vi "SpinProgramCheck.vi"() -> ()   [LabVIEW 2018]
uses:
  <instrlib>/Classes/SpinCoater/SpinCoater.lvclass
panel:
  out "Spin Program":dbl[][](array[numeric])
  in  "Time Start":dbl[unit]
  in  "Program":dbl[][](array[numeric])
  out "Init":bool
  in  "VISA resource name":refnum<visa-resource-name>
  in  "Cancel Button":bool
  out "Time Left":dbl
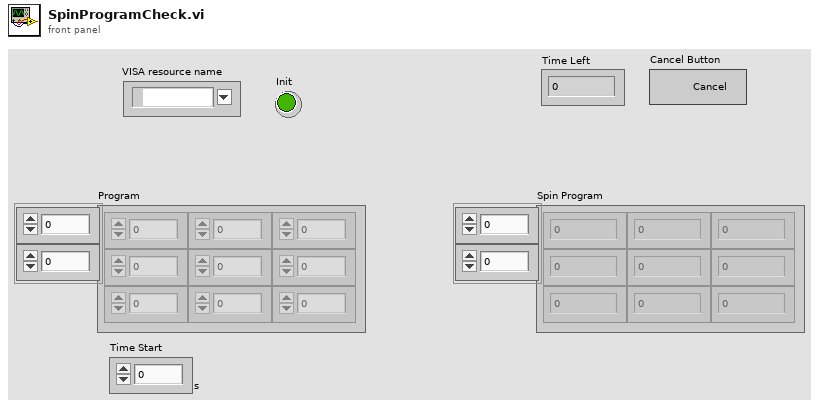
[diagram p1: front panel]
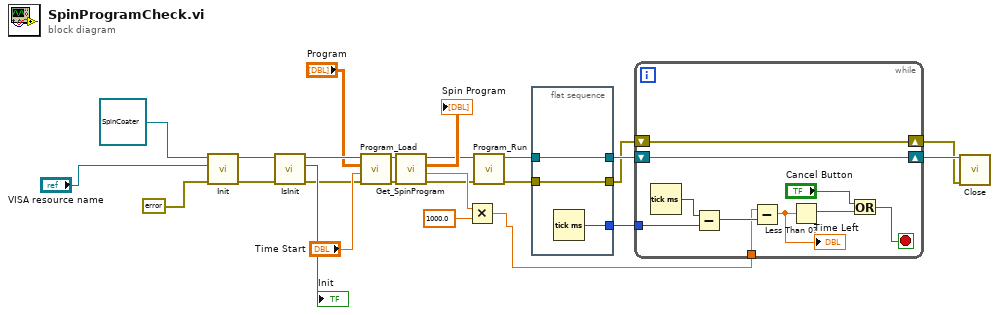
[diagram p0: block diagram]
diagram:
  n1 = call-dynamic "Init.vi"("error in (no error)"=errorcluster {"status"=FALSE, "code"=0, "source"=""}, "Variant"="VISA resource name", "SpinCoater in"=refnum<class "SpinCoater.lvclass"> refnum) -> ("error out"=w3:errorcluster, "SpinCoater out"=w21:refnum<class "SpinCoater.lvclass">)  [unwired: 7 in]
  n2 = call-dynamic "IsInit.vi"("error in (no error)"=w3, "SpinCoater in"=w21) -> ("error out"=w2:errorcluster, "Init"=→"Init":bool, "SpinCoater out"=w17:refnum<class "SpinCoater.lvclass">)  [unwired: 7 in]
  n3 = call-dynamic "Program_Load.vi"("error in (no error)"=w2, "Time Start"="Time Start", "Array"="Program", "SpinCoater in"=w17) -> ("error out"=w13:errorcluster, "SpinCoater out"=w12:refnum<class "SpinCoater.lvclass">)  [unwired: 6 in]
  n4 = call-dynamic "Get_SpinProgram.vi"("error in (no error)"=w13, "SpinCoater in"=w12) -> ("error out"=w1:errorcluster, "Spin Time (s)"=w24:dbl, "Spin Program"=→"Spin Program":dbl[][], "SpinCoater out"=w10:refnum<class "SpinCoater.lvclass">)  [unwired: 6 in]
  n5 = Multiply(x=w24, y=1000.0) -> (x*y=w22:dbl)
  n6 = call-dynamic "Program_Run.vi"("error in (no error)"=w1, "SpinCoater in"=w10) -> ("error out"=w9:errorcluster, "SpinCoater out"=w8:refnum<class "SpinCoater.lvclass">)  [unwired: 8 in]
  n7 = flat-sequence {
    tunnel: [w28] -> w25
    tunnel: w9 -> [w26]
    tunnel: w8 -> [w27]
    tunnel: [w27] -> w7
    tunnel: [w26] -> w6
    frame #0 {
      n8 = Tick Count (ms)() -> (millisecond timer value=w28:u32)
    }
  }
  n9 = while {
    tunnel: w25 -> [w37]
    tunnel: w22 -> [w35]
    shift-right: [w30] -> w4
    shift-left: w6 -> [w30]
    shift-right: [w29] -> w5
    shift-left: w7 -> [w29]
    stop <- w31 stop-if-true
    n10 = Tick Count (ms)() -> (millisecond timer value=w38:u32)
    n11 = Subtract(x=w38, y=w37) -> (x-y=w36:u32)
    n12 = Subtract(x=w35, y=w36) -> (x-y=w34:dbl)
    "Time Left" <- w34
    n13 = Less Than 0?(x=w34) -> (x < 0?=w33:bool)
    n14 = Or(x="Cancel Button", y=w33) -> (x .or. y?=w31:bool)
  }
  n15 = call-dynamic "Close.vi"("error in (no error)"=w4, "SpinCoater in"=w5) -> ()  [unwired: 8 in, 2 out]
